vi "MW_StartUp.vi"(6 "Delay Time (s)":dbl=0.1, 8 "error in (no error)":errorcluster, 10 "MW Power":T2 {"LO"."Power dBm" format="%.3p"; "Probe"."Power dBm" format="%.3p"}, 11 "MW Source In":T1) -> (0 "error out":errorcluster, 3 "MW Source Out":T1)   [LabVIEW 2016, in "Microwave Source.lvlib"]
uses:
  Microwave Source.lvlib
  MW_ctl_DeviceHandles..ctl
  MW_ctl_Powers.ctl
  MW_ctl_Power_single..ctl
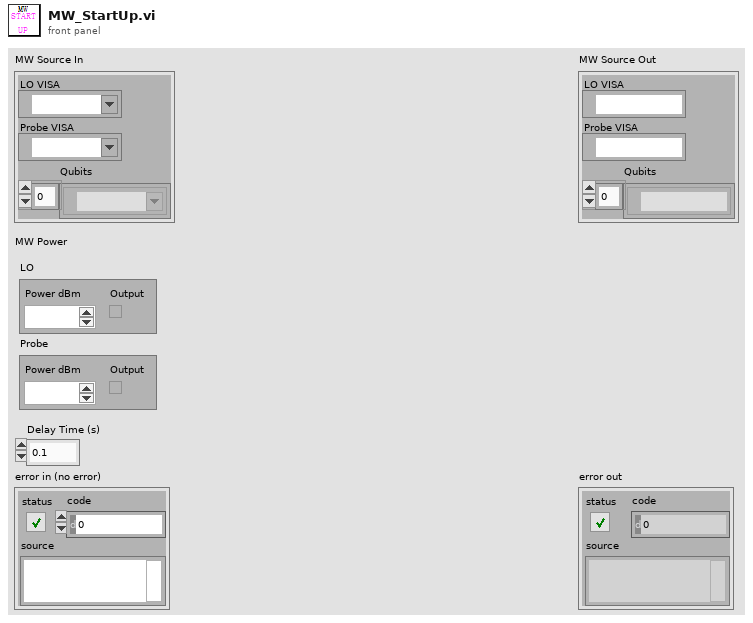
[diagram p1: front panel]
types:
  T1 = typedef "Microwave Source.lvlib/MW_ctl_DeviceHandles..ctl" = cluster{"LO VISA":refnum<visa-resource-name>, "Probe VISA":refnum<visa-resource-name>, "Qubits":refnum<visa-resource-name>[]}
  T2 = typedef "Microwave Source.lvlib/MW_ctl_Powers.ctl" = cluster{"LO":T3, "Probe":T3}
  T3 = typedef "Microwave Source.lvlib/MW_ctl_Power_single..ctl" = cluster{"Output":bool, "Power dBm":dbl}
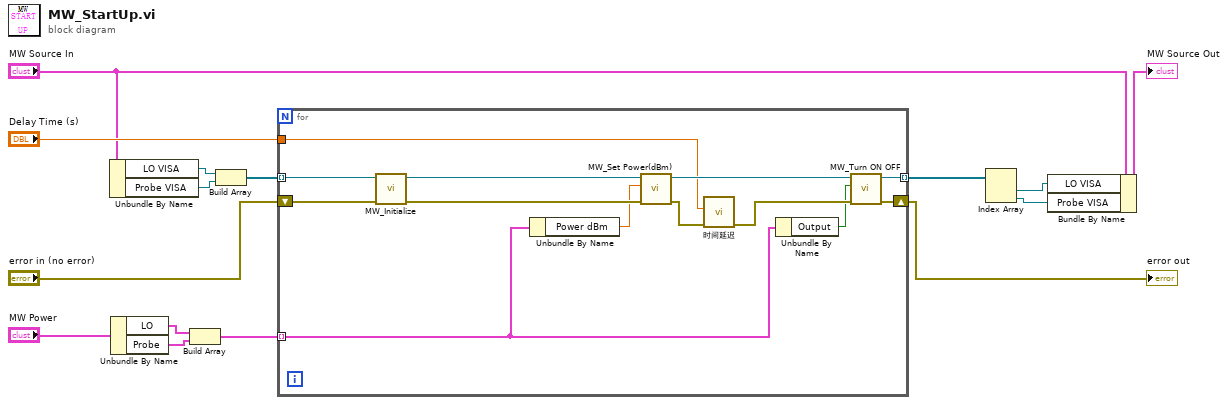
[diagram p0: block diagram]
diagram:
  n1 = Unbundle By Name("MW Source In") -> ("LO VISA"=w13:refnum<visa-resource-name>, "Probe VISA"=w14:refnum<visa-resource-name>)
  n2 = Unbundle By Name("MW Power") -> ("LO"=w9:T3, "Probe"=w8:T3)
  n3 = Build Array(w9, w8) -> (w7:T3[])
  n4 = Build Array(w13, w14) -> (w12:refnum<visa-resource-name>[])
  n5 = for {
    tunnel: "Delay Time (s)" -> [w23]
    tunnel: w12 -> [w22] mode=indexing
    shift-right: [w20] -> w5
    shift-left: "error in (no error)" -> [w21]
    tunnel: w7 -> [w18] mode=indexing
    tunnel: [w16] -> w4 mode=indexing
    n6 = call "MW_Initialize.vi"("error in (no error)"=w21, "VISA Refnum in"=w22) -> ("error out"=w28:errorcluster, "VISA Refnum out"=w27:refnum<visa-resource-name>)  [unwired: 8 in]
    n7 = Unbundle By Name(w18) -> ("Power dBm"=w19:dbl)
    n8 = call "MW_Set Power(dBm).vi"("错误输入（无错误）"=w28, "Power (dBm)"=w19, "VISA引用句柄输入"=w27) -> ("错误输出"=w24:errorcluster, "VISA引用句柄输出"=w26:refnum<visa-resource-name>)  [unwired: 6 in, 1 out]
    n9 = call "时间延迟"("error in (no error)"=w24, "Delay Time (s)"=w23) -> ("error out"=w25:errorcluster)  [unwired: 9 in]
    n10 = Unbundle By Name(w18) -> ("Output"=w17:bool)
    n11 = call "MW_Turn ON OFF.vi"("错误输入（无错误）"=w25, "start MW source?"=w17, "VISA引用句柄输入"=w26) -> ("错误输出"=w20:errorcluster, "VISA引用句柄输出"=w16:refnum<visa-resource-name>)  [unwired: 7 in]
  }
  "error out" <- w5
  n12 = Index Array(array=w4) -> (element #1=w2:refnum<visa-resource-name>, element #2=w1:refnum<visa-resource-name>)  [unwired: 2 in]
  n13 = Bundle By Name(cluster="MW Source In", "LO VISA"=w2, "Probe VISA"=w1) -> (→"MW Source Out":T1)
